vi "Get Nested Enq.vi"(8 "error in":errorcluster, 10 "Ident":string, 11 "Interactor in":refnum<class "Interactor.lvclass">) -> (0 "error out":errorcluster, 2 "Enq":refnum<class "Message Enqueuer.lvclass">, 3 "Interactor out":refnum<class "Interactor.lvclass">)   [LabVIEW 2024, in "Interactor.lvlib" / "Interactor.lvclass"]
uses:
  Interactor.lvclass
  <vilib>/ActorFramework/Message Enqueuer/Message Enqueuer.lvclass
  Interactor.lvclass/Interactor.ctl
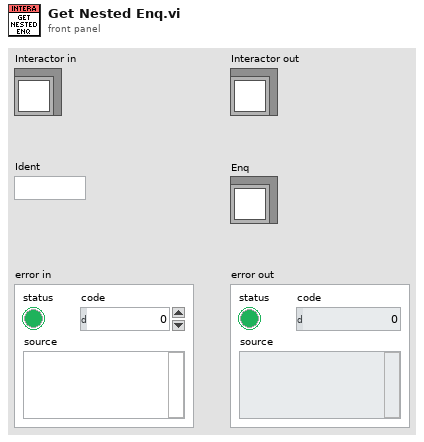
[diagram p1: front panel]
types:
  T1 = map{string, refnum<class "Message Enqueuer.lvclass">}
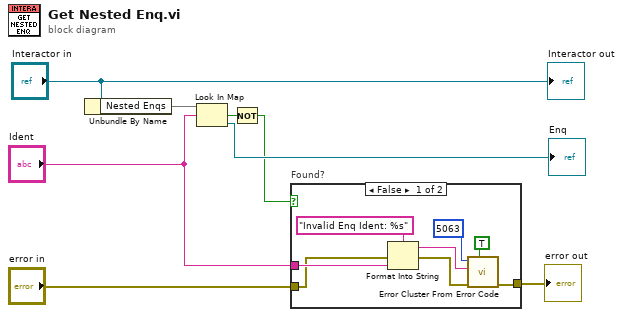
[diagram p0: block diagram]
diagram:
  n1 = Unbundle By Name("Interactor in") -> ("Nested Enqs"=w7:T1)
  n2 = Look In Map(map=w7, key="Ident") -> (key not found?=w6:bool, value=→"Enq":refnum<class "Message Enqueuer.lvclass">)  [unwired: 1 in]
  n3 = Not(x=w6) -> (.not. x?=w4:bool)
  n4 = case "Found?" shown="False" w4 {
    tunnel: "error in" -> [w10 w17]
    tunnel: [w16 w17] -> w2
    tunnel: "Ident" -> [w12 _]
    frame False {
      n5 = Format Into String(format string="Invalid Enq Ident: %s", error in=w10, w12) -> (resulting string=w11:string, error out=w9:errorcluster)  [unwired: 1 in]
      n6 = call <vilib>:"Error Cluster From Error Code.vi"("show call chain? (False)"=TRUE, "error in (no error)"=w9, "error message (\"\")"=w11, "error code (0)"=5063) -> ("error out"=w16:errorcluster)  [unwired: 5 in]
    }
    frame True {
    }
  }
  "error out" <- w2
  "Interactor out" <- "Interactor in"
